vi "HTTP Calendar.vi"(8 "error in":errorcluster) -> (0 "error out":errorcluster)   [LabVIEW 2020]
uses:
  System.Windows.Forms
panel:
  out "time lapsed":u32 format="%.0fms"
  in  "Password":string
  in  "User name":string="fedor@lanl.gov"
  out "IDs":string[](array[string])
  out "Names":string[](array[string])
  out "Elements count":i32
  in  "Stop Button":bool
  in  "urlString":string="https://users.magnet.fsu.edu/Users/LogIn.aspx"
  in  "WebBrowser":refnum<k24>(container)
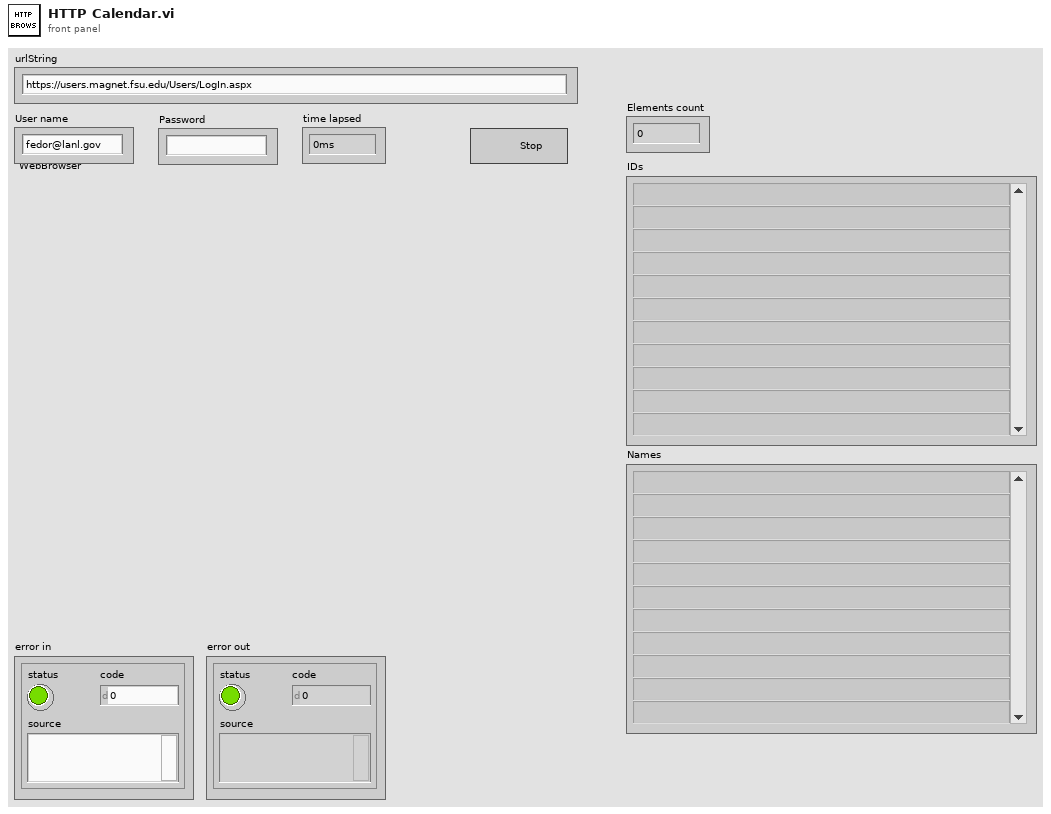
[diagram p1: front panel]
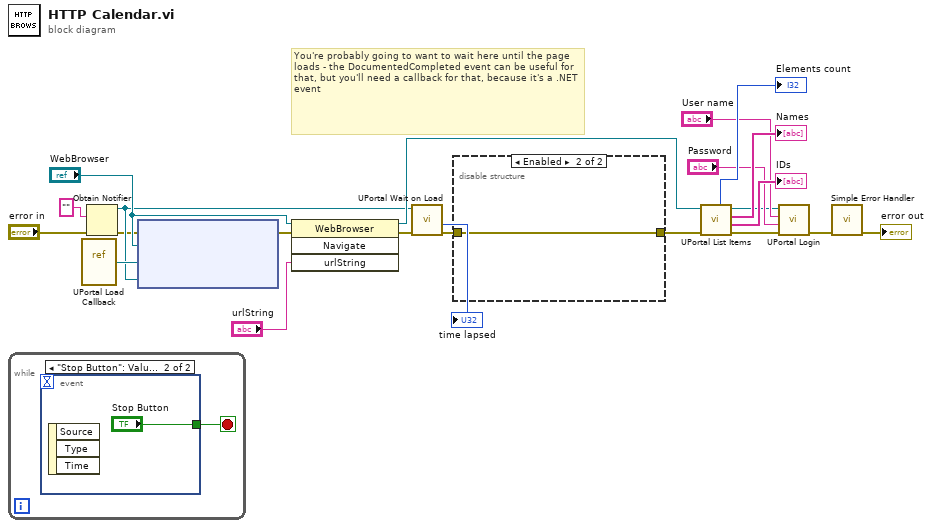
[diagram p0: block diagram]
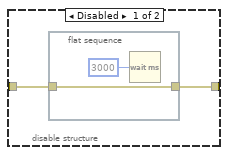
[diagram p2: hidden frame]
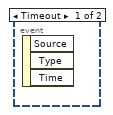
[diagram p3: hidden frame]
diagram:
  # "You're probably going to want to wait here until the page loads - the DocumentedCompleted event can be useful for that, but you'll need a callback for that, because it's a .NET event"
  n1 = while {
    stop <- w23 stop-if-true
    n2 = event shown="[1] \"Stop Button\": Value Change" {
      selector: _ -> [_ _]
      dyn-events: _ -> [_ _]
      timeout: _ -> [_ _]
      tunnel: [_ "Stop Button"] -> w23
      event Timeout {
        n3 = event-data() -> ()  [unwired: 1 in, 3 out]
      }
      event "Stop Button": Value Change {
        n4 = event-data() -> ()  [unwired: 1 in, 3 out]
      }
    }
  }
  n5 = vi-ref "UPortal Load Callback.vi"() -> ("vi reference"=w8:refnum<vi>)
  n6 = Obtain Notifier(notification data type="", error in (no error)="error in") -> (notifier out=w6:refnum<notifier>, error out=w4:errorcluster)  [unwired: 2 in, 1 out]
  n7 = node(w4, "WebBrowser", w8, w6) -> (w5:errorcluster)  [unwired: 1 in, 1 out]
  n8 = invoke class="WebBrowser" method="Navigate"(reference="WebBrowser", error in=w5, "urlString"="urlString") -> (reference out=w21:refnum<k24>, error out=w7:errorcluster)  [unwired: 1 in, 2 out]
  n9 = call "UPortal Wait on Load.vi"("error in"=w7, "notifier"=w6) -> ("error out"=w3:errorcluster, "time lapsed"=→"time lapsed":u32)  [unwired: 6 in, 2 out]
  n10 = disable-structure shown="Enabled" {
    disable-tunnel: w3 -> [w26 w29]
    disable-tunnel: [w25 w29] -> w2
    frame Disabled {
      n11 = flat-sequence {
        tunnel: w26 -> [w27]
        tunnel: [w27] -> w25
        frame #0 {
          n12 = Wait (ms)(milliseconds to wait=u32 3000) -> ()  [unwired: 1 out]
        }
      }
    }
    frame Enabled {
    }
  }
  n13 = call "UPortal List Items.vi"("error in (no error)"=w2, ".NET Refnum in"=w21) -> ("error out"=w12:errorcluster, "Array"=→"IDs":string[], "Array 2"=→"Names":string[], ".NET Refnum out"=w13:refnum<k24>, "Count"=→"Elements count":i32)  [unwired: 5 in]
  n14 = call "UPortal Login.vi"("error in"=w12, "Password"="Password", "User name"="User name", "Browser reference"=w13) -> ("error out"=w11:errorcluster)  [unwired: 6 in, 1 out]
  n15 = call <vilib>:"Simple Error Handler.vi"("error in (no error)"=w11) -> ("error out"=→"error out":errorcluster)  [unwired: 4 in, 4 out]
